vi "BuildSunCheckSum (SubVI).vi"(10 "Array in":u16[](array[numeric])) -> (0 "CheckSum DataB":u16 format="%.0x", 1 "Buff Out":u8[](array[numeric]), 2 "ExpectedCheckSum":string, 3 "ExpectedCheckSum":u16)   [LabVIEW 2017]
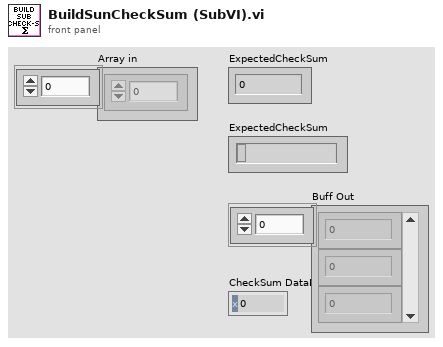
[diagram p1: front panel]
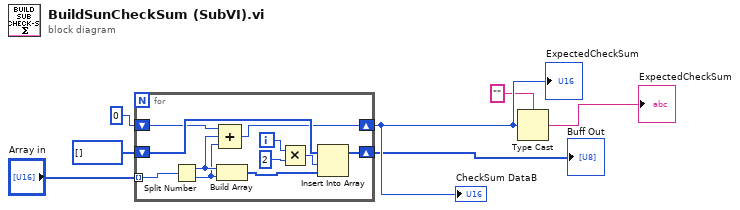
[diagram p0: block diagram]
diagram:
  n1 = for {
    tunnel: "Array in" -> [w18] mode=indexing
    shift-right: [w13] -> w3
    shift-left: u8[] [] -> [w12]
    shift-right: [w10] -> w7
    shift-left: u16 0 -> [w11]
    i -> [w17]
    n2 = Split Number(x=w18) -> (hi(x)=w9:u8, lo(x)=w8:u8)
    n3 = Build Array(w9, w8) -> (w15:u8[])
    n4 = Compound Arithmetic op=ADD(w11, w9, w8) -> (w10:u16)
    n5 = Multiply(x=w17, y=2) -> (x*y=w14:i32)
    n6 = Insert Into Array(array=w12, index=w14, new element=w15) -> (w13:u8[])
  }
  "CheckSum DataB" <- w7
  "ExpectedCheckSum" <- w7
  "Buff Out" <- w3
  n7 = Type Cast(type="", x=w7) -> (*(type *) &x=→"ExpectedCheckSum":string)
